vi "Process_data.vi"(0 "PWA Binary":i16[][](array[numeric]), 1 "Analogue Binary":i16[][](array[numeric]), 2 "LDA Binary output":u16[][](array[numeric]), 3 "Analogue volts":dbl[][](array[numeric]) format="%.2f", 4 "Measurement top level?":bool, 5 "Block Timings":T1={"Started"=0.0, "Ended"=0.0, "Analogue Frequency Hz"=1000.0} {"Analogue Frequency Hz" format="%.2f"}) -> (6 "Vel stat display":string[][](table), 7 "First Plot data":cluster{"Xo":dbl, "Delta X":dbl, dbl[]}[](array[cluster]) {"?" format="%.2f"; "Delta X" format="%.2f"; "Xo" format="%.2f"}, 8 "Second Plot data":cluster{"Xo":dbl, "Delta X":dbl, dbl[]}[](array[cluster]) {"?" format="%.2f"; "Delta X" format="%.2f"; "Xo" format="%.2f"}, 9 "Max Measurement time up":bool)   [LabVIEW 2011]
uses:
  Controls/Block_start_and_end.ctl
  Controls/Correlation_cluster.ctl
  Controls/Inst_type.ctl
  Controls/Instrument_Array.ctl
  Globals/Meas_global.vi
  Globals/LDA_meas_global_1.vi
  Acquisition/PWA/PWAtasksGLOBAL.vi
  Globals/Dynamic_call_global.ph.vi
  Globals/Plug_in_data_global.vi
  <vilib>/Analysis/NI_AALBase.lvlib
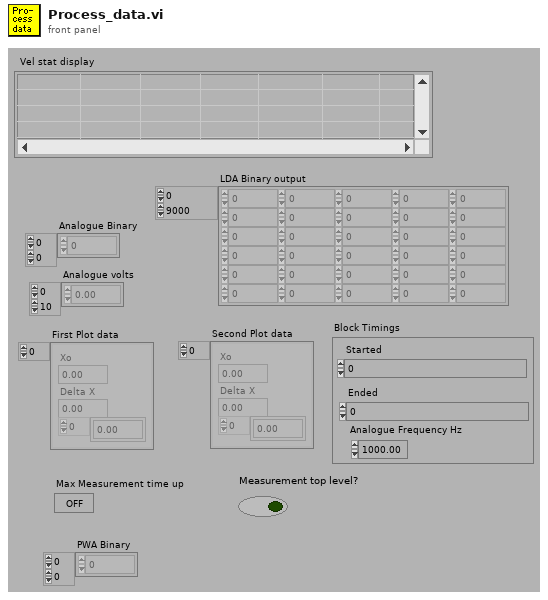
[diagram p1: front panel]
types:
  T1 = typedef "Block_start_and_end.ctl" = cluster{"Started":dbl, "Ended":dbl, "Analogue Frequency Hz":dbl}
  T2 = typedef "PWA_Data.ctl" = enum16{"No PWA Data", "One Ch PWA"}
  T3 = typedef "BSA_Type.ctl" = enum16{"57N11", "BSA F60"}
  T4 = typedef "Correlation_cluster.ctl" = cluster{"U inst":string, "W inst":string, "uw":dbl, "uw/u'w'":dbl, "u^2w":dbl, "uw^2":dbl, "uw^3":dbl, "u^3w":dbl, "u^2w^2":dbl}
  T5 = typedef "Inst_type.ctl" = enum16{"Propeller anemometer", "Raw voltage", "Pressure Transducer", "Pitot-static tube", "Preston tube", "Hot wire", "Cross wire 1", "Cross wire 2", "Generic Linear", "Generic Polynomial", "Generic BackPoly", "Fast FID", "Thermocouple", "Cold wire", "Pulsed Wire", "LDA Vel", "LDA Tran time", "LDA Arr time"}
  T6 = typedef "Instrument_Array.ctl" = enum16{"PWA", "LDA", "Analogue"}
  T7 = typedef "Analysis_info_cluster.ctl" = cluster{"Colour":u32, "Inst type":T5, "Inst name":string, "Symbol":string, "Code name":string, "Extra Info":string, "Inst Array":T6, "Index":i32, "Voltage Index":i32, "Extra Titles":string[], "Extra Values":string[], "Eng Values":dbl[], "Time (ms)":dbl[], "TT / Voltage":dbl[], "U":dbl, "u^2":dbl, "u^3":dbl, "u^4":dbl, "Skew_u":dbl, "Kurt_u":dbl, "Mean % Err":dbl, "% u'/U":dbl}
  T8 = typedef "Post_Process.ctl" = enum16{"Take New Data", "Post Process Raw Data File"}
  T9 = typedef "Graph_Type.ctl" = enum16{"Show no graph", "Voltage trace", "Velocity trace", "Vel histogram", "Spectrum", "f.E(f) v Log f", "Auto-Corr"}
  T10 = cluster{"Plot 1":u16, "Plot 2":u16, "Save graph":u16, "Plot Type":T9}
  T11 = typedef "Board_Types.ctl" = enum16{"Simulate", "Local ADAM", "Server ADAM", "NI-DAQmx", "NI-DAQmxBase", "ADC488", "DT LV-link"}
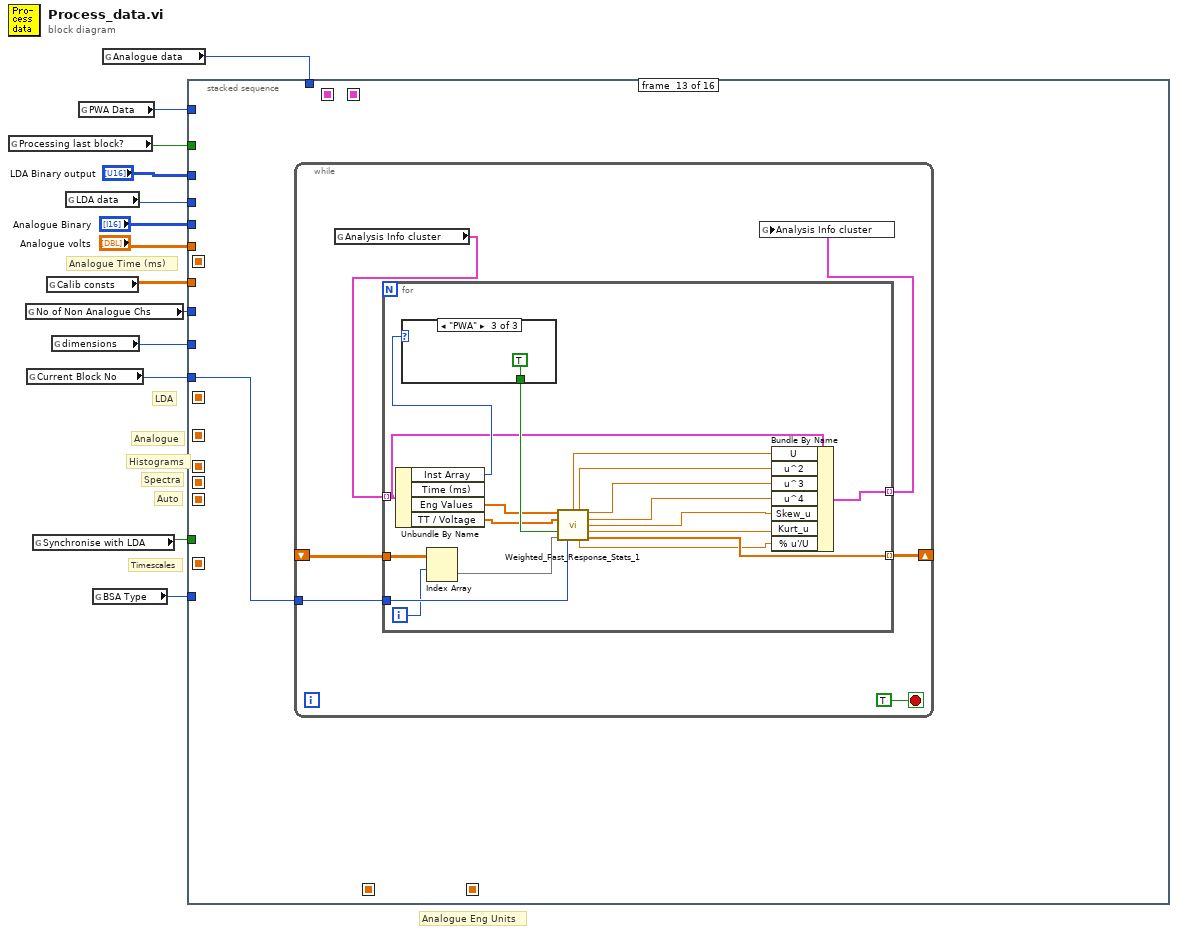
[diagram p0: block diagram]
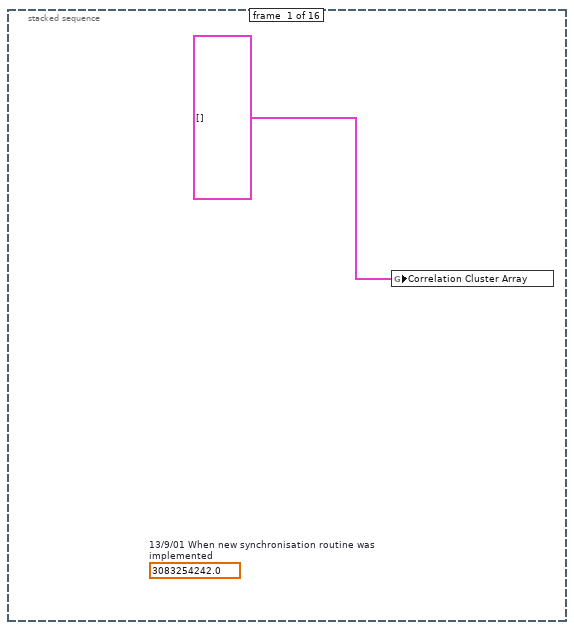
[diagram p2: hidden frame]
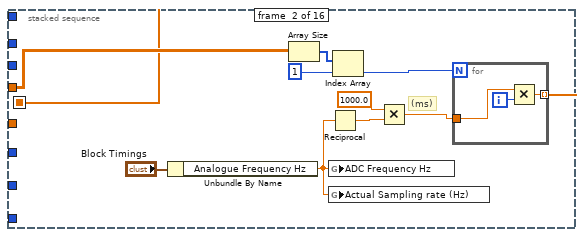
[diagram p3: hidden frame]
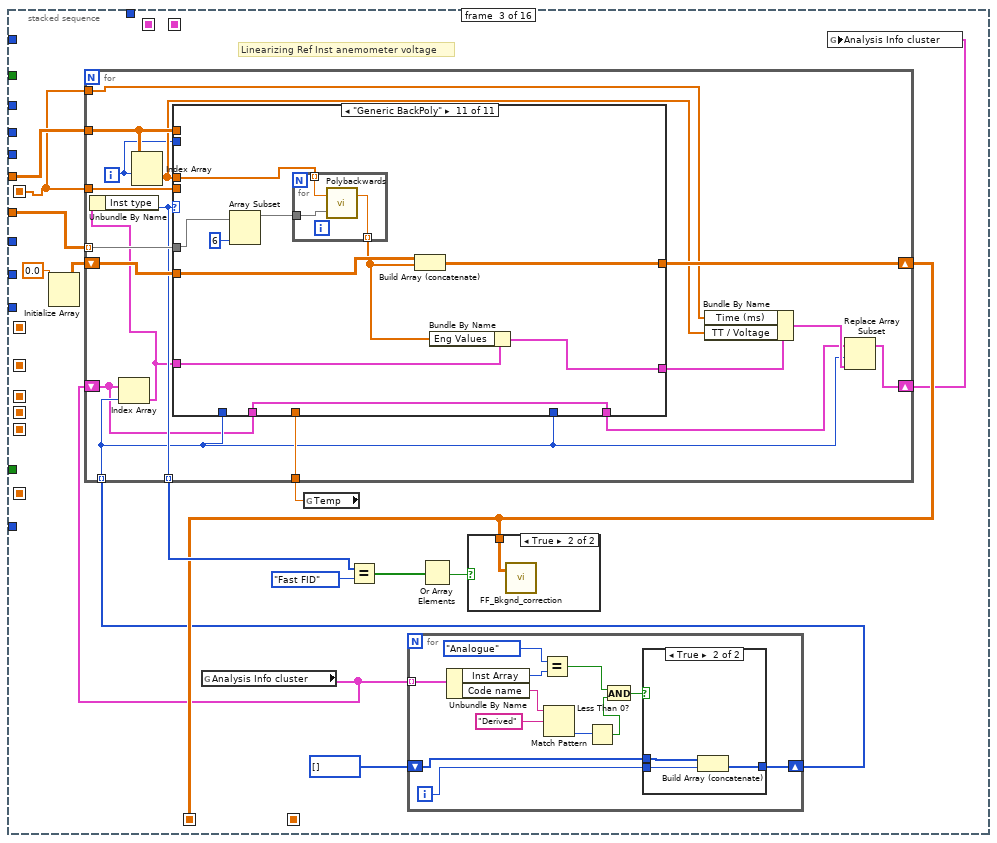
[diagram p4: hidden frame]
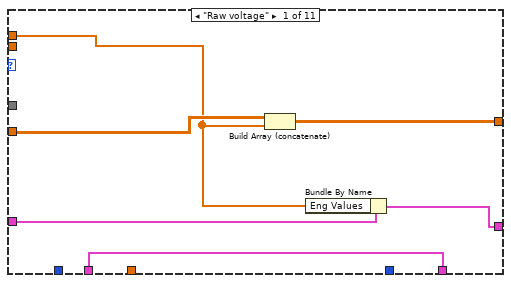
[diagram p7: hidden frame]
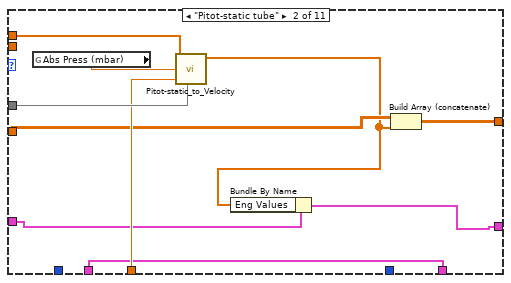
[diagram p8: hidden frame]
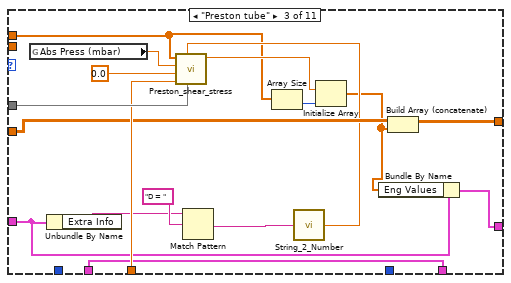
[diagram p9: hidden frame]
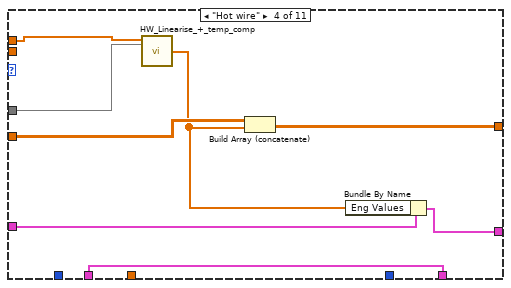
[diagram p10: hidden frame]
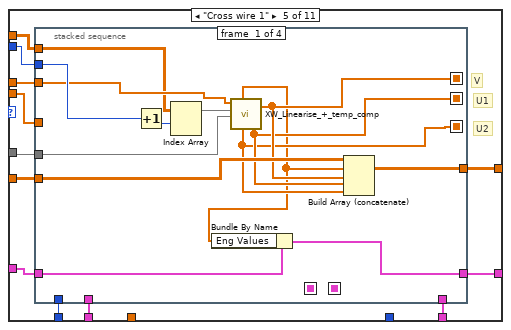
[diagram p11: hidden frame]
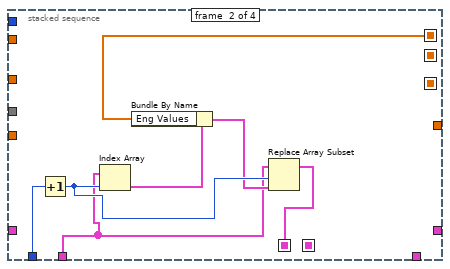
[diagram p12: hidden frame]
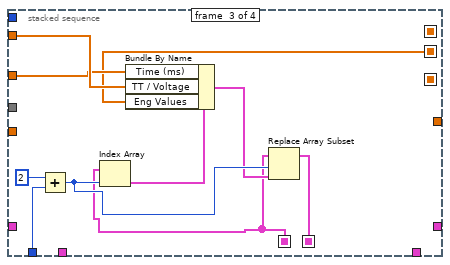
[diagram p13: hidden frame]
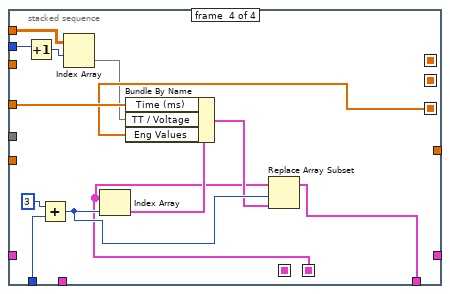
[diagram p14: hidden frame]
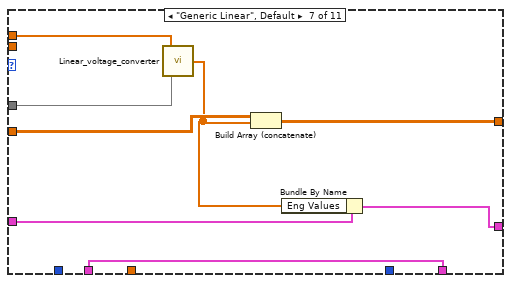
[diagram p16: hidden frame]
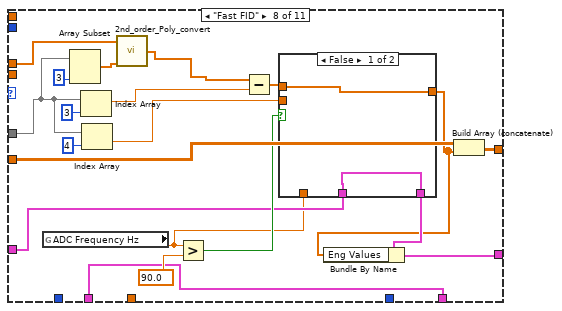
[diagram p17: hidden frame]
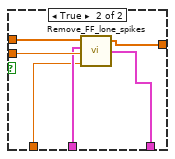
[diagram p18: hidden frame]
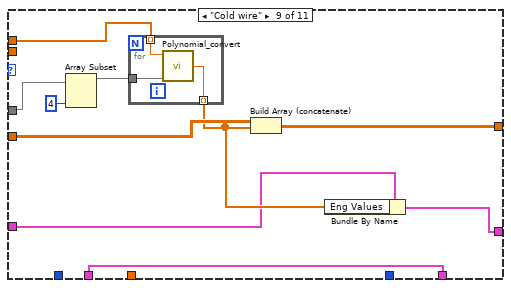
[diagram p19: hidden frame]
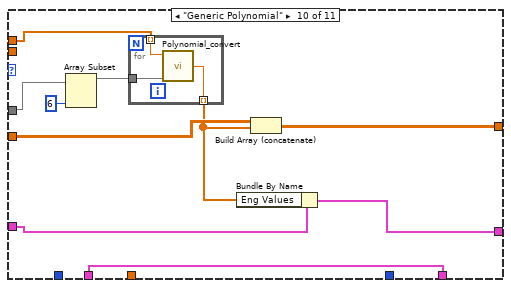
[diagram p20: hidden frame]
diagram:
  # "Analogue Time (ms)"
  # "Timescales"
  # "LDA"
  # "Auto"
  # "Spectra"
  # "Histograms"
  # "Analogue Eng Units"
  # "Analogue"
  n1 = global read "Meas_global.vi" "Processing last block?"() -> (w9:bool)
  n2 = global read "Meas_global.vi" "No of Non Analogue Chs"() -> (w5:i32)
  n3 = global read "Meas_global.vi" "Current Block No"() -> (w10:i32)
  n4 = global read "Meas_global.vi" "Synchronise with LDA"() -> (w4:bool)
  n5 = global read "Meas_global.vi" "Calib consts"() -> (w3:dbl[][])
  n6 = global read "Meas_global.vi" "dimensions"() -> (w13:enum16{"1D", "2D"})
  n7 = global read "Meas_global.vi" "LDA data"() -> (w12:enum16{"No LDA data", "Take LDA data"})
  n8 = global read "Meas_global.vi" "PWA Data"() -> (w2:T2)
  n9 = global read "LDA_meas_global_1.vi" "BSA Type"() -> (w1:T3)
  n10 = global read "Meas_global.vi" "Analogue data"() -> (w11:enum16{"No Analogue data", "Take Analogue data"})
  n11 = stacked-sequence {
    seq-local: [_ _ _ _ w278 _ _ _ _ _ _ _ _ _ _ _] -> [_ _ _ _ _ _ w545 w558 w566 w581 w592 w611 _ w644 _ _]
    seq-local: [_ _ _ w253 _ _ _ _ _ _ _ _ _ _ _ _] -> [_ _ _ _ w280 _ _ _ _ _ _ _ _ _ _ _]
    seq-local: [_ _ _ _ _ _ w544 _ _ _ _ _ _ _ _ _] -> [_ _ _ _ _ _ _ _ _ w580 _ _ _ _ w687 _]
    seq-local: [_ _ _ _ _ _ _ w557 _ _ _ _ _ _ _ _] -> [_ _ _ _ _ _ _ _ _ w579 _ _ _ _ _ _]
    seq-local: [_ _ _ _ _ _ _ _ w565 _ _ _ _ _ _ _] -> [_ _ _ _ _ _ _ _ _ w578 w599 _ _ _ _ _]
    seq-local: [_ _ _ _ _ _ _ _ _ w573 _ _ _ _ _ _] -> [_ _ _ _ _ _ _ _ _ _ _ _ _ w650 _ _]
    seq-local: [_ _ _ _ _ _ _ _ _ w572 _ _ _ _ _ _] -> [_ _ _ _ _ _ _ _ _ _ _ _ _ w649 _ _]
    seq-local: [_ _ _ _ w275 _ _ _ _ _ _ _ _ _ _ _] -> [_ _ _ _ _ _ w546 _ _ w571 _ w612 _ w645 _ w700]
    seq-local: [_ _ _ _ _ _ _ _ _ _ w585 _ _ _ _ _] -> [_ _ _ _ _ _ _ _ _ _ _ w609 _ _ _ w699]
    seq-local: [_ _ w33 _ _ _ _ _ _ _ _ _ _ _ _ _] -> [_ _ _ w252 _ _ _ _ _ _ _ _ _ _ _ _]
    seq-local: [_ w18 _ _ _ _ _ _ _ _ _ _ _ _ _ _] -> [_ _ w28 _ _ _ _ _ _ _ _ _ _ _ _ _]
    tunnel: w10 -> [_ _ _ _ _ w444 _ _ _ _ _ _ w613 _ _ _]
    tunnel: w13 -> [_ _ _ _ w282 _ _ _ _ _ _ _ _ _ _ _]
    tunnel: w12 -> [_ _ _ _ w281 _ _ _ _ _ _ _ _ _ _ _]
    tunnel: w11 -> [_ _ _ _ w279 _ _ _ _ _ _ _ _ _ _ _]
    tunnel: w9 -> [_ _ _ _ _ _ _ _ _ _ _ _ _ _ w688 _]
    tunnel: "LDA Binary output" -> [_ _ _ _ w277 _ _ _ _ _ _ _ _ w648 _ _]
    tunnel: "Analogue Binary" -> [_ _ _ _ w272 _ _ _ _ _ _ _ _ w647 w686 _]
    tunnel: "Analogue volts" -> [_ w23 w39 _ w271 _ _ _ _ w570 _ _ _ w646 w681 _]
    tunnel: w5 -> [_ _ _ _ _ _ _ _ _ _ _ _ _ _ _ _]
    tunnel: w4 -> [_ _ _ _ w276 _ _ _ _ _ _ _ _ _ _ _]
    tunnel: w3 -> [_ _ w38 _ _ _ _ _ _ _ _ _ _ _ _ _]
    tunnel: w2 -> [_ _ _ _ _ w448 _ _ _ _ _ _ _ _ _ _]
    tunnel: w1 -> [_ _ _ _ w270 _ _ _ _ _ _ _ _ _ _ _]
    frame #0 {
      (unwired) 3083254242.0  # 13/9/01 When new synchronisation routine was implemented
      n12 = global write "Meas_global.vi" "Correlation Cluster Array"(T4[] [] ("Correlation Cluster Array")) -> ()
    }
    frame #1 {
      # "(ms)"
      n13 = Unbundle By Name("Block Timings") -> ("Analogue Frequency Hz"=w19:dbl)
      n14 = Array Size(array=w23) -> (size(s)=w22:i32[])
      n15 = global write "LDA_meas_global_1.vi" "ADC Frequency Hz"(w19) -> ()
      n16 = global write "Meas_global.vi" "Actual Sampling rate (Hz)"(w19) -> ()
      n17 = Reciprocal(x=w19) -> (1/x=w17:dbl)
      n18 = Index Array(array=w22, index=1) -> (element=w20:i32)
      n19 = Multiply(x=1000.0, y=w17) -> (x*y=w15:dbl)
      n20 = for {
        N: w20 -> [_]
        tunnel: w15 -> [w26]
        tunnel: [w25] -> w18 mode=indexing
        i -> [w27]
        n21 = Multiply(x=w26, y=w27) -> (x*y=w25:dbl)
      }
    }
    frame #2 {
      # "Linearizing Ref Inst anemometer voltage"
      n22 = Initialize Array(0.0) -> (w41:dbl[][])  [unwired: 2 out]
      n23 = global read "Meas_global.vi" "Analysis Info cluster"() -> (w30:T7[])
      n24 = global read "Meas_global.vi" "Temp"() -> (w40:dbl)
      n25 = for {
        tunnel: w30 -> [w46] mode=indexing
        shift-right: [w43] -> w29
        shift-left: i32[] [] -> [w44]
        i -> [w45]
        n26 = Unbundle By Name(w46) -> ("Inst Array"=w54:T6, "Code name"=w52:string)
        n27 = Equal?(x=Instrument_Array."Analogue" ("Inst Array"), y=w54) -> (x = y?=w48:bool)
        n28 = Match Pattern(string=w52, regular expression="Derived") -> (offset past match=w50:i32)  [unwired: 4 out]
        n29 = Less Than 0?(x=w50) -> (x < 0?=w49:bool)
        n30 = And(x=w48, y=w49) -> (x .and. y?=w47:bool)
        n31 = case shown="True" w47 {
          tunnel: w45 -> [_ w58]
          tunnel: w44 -> [w55 w57]
          tunnel: [w55 w56] -> w43
          frame False {
          }
          frame True {
            n32 = Build Array (concatenate)(w57, w58) -> (w56:i32[])
          }
        }
      }
      n33 = for {
        tunnel: w39 -> [w65]
        tunnel: w38 -> [w76] mode=indexing
        shift-right: [w74] -> w33
        shift-left: w41 -> [w75]
        tunnel: w40 -> [w73]
        tunnel: [w72] -> w36 mode=indexing
        tunnel: w29 -> [w62] mode=indexing
        shift-right: [w70] -> w32
        shift-left: w30 -> [w61]
        tunnel: w28 -> [w69]
        tunnel: w28 -> [w66]
        i -> [w63]
        n34 = Index Array(array=w61, index=w62) -> (element=w71:T7)
        n35 = Unbundle By Name(w71) -> ("Inst type"=w72:T5)
        n36 = Index Array(array=w65, index (row)=w63) -> (element=w64:dbl[])  [unwired: 1 in]
        n37 = case shown="\"Generic BackPoly\"" w72 {
          tunnel: w76 -> [_ w92 w109 w117 w126 _ w184 w196 w220 w233 w246]
          tunnel: w73 -> [_ w91 w108 _ _ _ _ _ _ _ _]
          tunnel: w63 -> [_ _ _ _ w129 _ _ _ _ _ _]
          tunnel: w65 -> [_ _ _ _ w124 _ _ _ _ _ _]
          tunnel: w75 -> [w82 w90 w107 w115 w128 w176 w182 w204 w221 w234 w247]
          tunnel: [w81 w89 w106 w116 w127 w176 w183 w191 w222 w235 w248] -> w74
          tunnel: w71 -> [w80 w85 w96 w112 w123 w175 w180 w192 w215 w228 w241]
          tunnel: w62 -> [_ _ _ _ _ _ _ _ _ _ _]
          tunnel: [w79 w84 w95 w113 w122 w175 w179 w187 w214 w226 w240] -> w68
          tunnel: w69 -> [_ _ _ _ w119 _ _ _ _ _ _]
          tunnel: w64 -> [w77 w87 w93 w110 w125 _ w177 w185 w213 w229 w242]
          tunnel: w62 -> [_ _ _ _ w121 _ _ _ _ _ _]
          tunnel: w61 -> [w78 w86 w97 w114 w120 w174 w181 w189 w217 w230 w243]
          tunnel: [w78 w86 w97 w114 w118 w174 w181 w189 w217 w230 w243] -> w60
          frame "Raw voltage" {
            n38 = Build Array (concatenate)(w82, w77) -> (w81:dbl[][])
            n39 = Bundle By Name(cluster=w80, "Eng Values"=w77) -> (w79:T7)
          }
          frame "Pitot-static tube" {
            n40 = global read "Meas_global.vi" "Abs Press (mbar)"() -> (w88:dbl)
            n41 = call "Pitot-static_to_Velocity.vi"("Pressure Trans voltage"=w87, "Atmos Press mbar  (1000)"=w88, "Temp  C  (20)"=w91, "Pressure Trans Calib const"=w92) -> ("Velocity (m/s)"=w83:dbl[])  [unwired: 1 in, 3 out]
            n42 = Bundle By Name(cluster=w85, "Eng Values"=w83) -> (w84:T7)
            n43 = Build Array (concatenate)(w90, w83) -> (w89:dbl[][])
          }
          frame "Preston tube" {
            n44 = global read "Meas_global.vi" "Abs Press (mbar)"() -> (w105:dbl)
            n45 = Unbundle By Name(w96) -> ("Extra Info"=w102:string)
            n46 = Match Pattern(string=w102, regular expression="D = " ("String to match")) -> (after substring=w103:string)  [unwired: 4 out]
            n47 = Array Size(array=w93) -> (size(s)=w99:i32)
            n48 = call "String_2_Number.vi"("Value"=w103) -> ("Numeric"=w101:dbl)
            n49 = call "Preston_shear_stress.vi"("Calib. consts"=w109, "Diam. (mm)"=w101, "Temp (C)"=w108, "Static gauge head mm H2O"=0.0 ("Static gauge press mm H2O"), "Atmos. pressure (mbars)"=w105, "Pressure transducer voltages"=w93) -> ("Mean shear stress (Pa)"=w98:dbl)  [unwired: 1 in, 3 out]
            n50 = Initialize Array(w98, w99) -> (w94:dbl[])
            n51 = Bundle By Name(cluster=w96, "Eng Values"=w94) -> (w95:T7)
            n52 = Build Array (concatenate)(w107, w94) -> (w106:dbl[][])
          }
          frame "Hot wire" {
            n53 = call "HW_Linearise_+_temp_comp.vi"("Caib const"=w117, "HW voltage"=w110) -> ("Velocity"=w111:dbl[])  [unwired: 3 in, 1 out]
            n54 = Build Array (concatenate)(w115, w111) -> (w116:dbl[][])
            n55 = Bundle By Name(cluster=w112, "Eng Values"=w111) -> (w113:T7)
          }
          frame "Cross wire 1" {
            # "U2"
            # "U1"
            # "V"
            n56 = stacked-sequence {
              seq-local: [w135 _ _ _] -> [_ w149 _ _]
              seq-local: [w134 _ _ _] -> [_ _ w151 _]
              seq-local: [w133 _ _ _] -> [_ _ _ w165]
              seq-local: [_ w144 _ _] -> [_ _ w154 _]
              seq-local: [_ _ w153 _] -> [_ _ _ w168]
              tunnel: w129 -> [w143 _ _ w164]
              tunnel: w128 -> [w141 _ _ _]
              tunnel: [w140 _ _ _] -> w127
              tunnel: w126 -> [w138 _ _ _]
              tunnel: w125 -> [w137 _ w159 _]
              tunnel: w124 -> [w136 _ _ w162]
              tunnel: w123 -> [w132 _ _ _]
              tunnel: [w130 _ _ _] -> w122
              tunnel: w121 -> [_ w150 w160 w173]
              tunnel: w120 -> [_ w145 _ _]
              tunnel: w119 -> [_ _ w158 w172]
              tunnel: [_ _ _ w167] -> w118
              frame #0 {
                n57 = Increment(x=w143) -> (x+1=w142:i32)
                n58 = Index Array(array=w136, index (row)=w142) -> (element=w139:dbl[])  [unwired: 1 in]
                n59 = call "XW_Linearise_+_temp_comp.vi"("Calib const"=w138, "XW2 voltage"=w139, "XW1 voltage"=w137) -> ("U1"=w134:dbl[], "V"=w135:dbl[], "U2"=w133:dbl[], "U"=w131:dbl[])  [unwired: 1 in]
                n60 = Bundle By Name(cluster=w132, "Eng Values"=w131) -> (w130:T7)
                n61 = Build Array (concatenate)(w141, w131, w135, w134, w133) -> (w140:dbl[][])
              }
              frame #1 {
                n62 = Increment(x=w150) -> (x+1=w147:i32)
                n63 = Index Array(array=w145, index=w147) -> (element=w148:T7)
                n64 = Bundle By Name(cluster=w148, "Eng Values"=w149) -> (w146:T7)
                n65 = Replace Array Subset(array=w145, new element=w146, index=w147) -> (w144:T7[])
              }
              frame #2 {
                n66 = Add(x=2, y=w160) -> (x+y=w156:i32)
                n67 = Index Array(array=w154, index=w156) -> (element=w157:T7)
                n68 = Bundle By Name(cluster=w157, "Time (ms)"=w158, "TT / Voltage"=w159, "Eng Values"=w151) -> (w155:T7)
                n69 = Replace Array Subset(array=w154, new element=w155, index=w156) -> (w153:T7[])
              }
              frame #3 {
                n70 = Increment(x=w164) -> (x+1=w163:i32)
                n71 = Add(x=3, y=w173) -> (x+y=w170:i32)
                n72 = Index Array(array=w162, index (row)=w163) -> (element=w161:dbl[])  [unwired: 1 in]
                n73 = Index Array(array=w168, index=w170) -> (element=w171:T7)
                n74 = Bundle By Name(cluster=w171, "Time (ms)"=w172, "TT / Voltage"=w161, "Eng Values"=w165) -> (w169:T7)
                n75 = Replace Array Subset(array=w168, new element=w169, index=w170) -> (w167:T7[])
              }
            }
          }
          frame "Cross wire 2" {
          }
          frame "Generic Linear", Default {
            n76 = call "Linear_voltage_converter.vi"("Caib const A,B"=w184, "Voltage array"=w177) -> ("Converted array"=w178:dbl[])
            n77 = Build Array (concatenate)(w182, w178) -> (w183:dbl[][])
            n78 = Bundle By Name(cluster=w180, "Eng Values"=w178) -> (w179:T7)
          }
          frame "Fast FID" {
            n79 = global read "LDA_meas_global_1.vi" "ADC Frequency Hz"() -> (w190:dbl)
            n80 = Array Subset(array=w196, length=3) -> (w195:dbl[])  [unwired: 1 in]
            n81 = Index Array(array=w196, index=3) -> (element=w202:dbl)
            n82 = Index Array(array=w196, index=4) -> (element=w198:dbl)
            n83 = call "2nd_order_Poly_convert.vi"("Calib constants"=w195, "Voltage"=w185) -> ("Eng Values"=w194:dbl[])  [unwired: 4 out]
            n84 = Greater?(x=w190, y=90.0) -> (0:w193:bool)
            n85 = Subtract(x=w194, y=w202) -> (x-y=w201:dbl[])
            n86 = case shown="False" w193 {
              tunnel: w201 -> [w206 w212]
              tunnel: [w206 w211] -> w186
              tunnel: w198 -> [_ w210]
              tunnel: w192 -> [w205 w209]
              tunnel: w190 -> [_ w208]
              tunnel: [w205 w207] -> w188
              frame False {
              }
              frame True {
                n87 = call "Remove_FF_lone_spikes.vi"("ADC Frequency Hz"=w208, "Bkgnd variance"=w210, "Analysis Info cluster"=w209, "Time Trace"=w212) -> ("Analysis Info cluster out"=w207:T7, "Filtered Time Trace"=w211:dbl[])  [unwired: 1 out]
              }
            }
            n88 = Bundle By Name(cluster=w188, "Eng Values"=w186) -> (w187:T7)
            n89 = Build Array (concatenate)(w204, w186) -> (w191:dbl[][])
          }
          frame "Cold wire" {
            n90 = Array Subset(array=w220, length=4) -> (w219:dbl[])  [unwired: 1 in]
            n91 = for {
              tunnel: w219 -> [w225]
              tunnel: w213 -> [w224] mode=indexing
              tunnel: [w223] -> w216 mode=indexing
              n92 = call "Polynomial_convert.vi"("Calib constants"=w225, "Voltage"=w224) -> ("Eng Values"=w223:dbl)  [unwired: 4 out]
            }
            n93 = Build Array (concatenate)(w221, w216) -> (w222:dbl[][])
            n94 = Bundle By Name(cluster=w215, "Eng Values"=w216) -> (w214:T7)
          }
          frame "Generic Polynomial" {
            n95 = Array Subset(array=w233, length=6) -> (w232:dbl[])  [unwired: 1 in]
            n96 = for {
              tunnel: w232 -> [w238]
              tunnel: w229 -> [w237] mode=indexing
              tunnel: [w236] -> w227 mode=indexing
              n97 = call "Polynomial_convert.vi"("Calib constants"=w238, "Voltage"=w237) -> ("Eng Values"=w236:dbl)  [unwired: 4 out]
            }
            n98 = Bundle By Name(cluster=w228, "Eng Values"=w227) -> (w226:T7)
            n99 = Build Array (concatenate)(w234, w227) -> (w235:dbl[][])
          }
          frame "Generic BackPoly" {
            n100 = Array Subset(array=w246, length=6) -> (w245:dbl[])  [unwired: 1 in]
            n101 = for {
              tunnel: w245 -> [w251]
              tunnel: w242 -> [w250] mode=indexing
              tunnel: [w249] -> w239 mode=indexing
              n102 = call "Polybackwards.vi"("Coefficients"=w251, "Y input"=w250) -> ("X output"=w249:dbl)  [unwired: 1 out]
            }
            n103 = Build Array (concatenate)(w247, w239) -> (w248:dbl[][])
            n104 = Bundle By Name(cluster=w241, "Eng Values"=w239) -> (w240:T7)
          }
        }
        n105 = Bundle By Name(cluster=w68, "Time (ms)"=w66, "TT / Voltage"=w64) -> (w67:T7)
        n106 = Replace Array Subset(array=w60, new element=w67, index=w62) -> (w70:T7[])
      }
      n107 = Equal?(x=w36, y=Inst_type."Fast FID" ("Inst type")) -> (x = y?=w35:bool[])
      n108 = Or Array Elements(Boolean array=w35) -> (logical OR=w34:bool)
      n109 = case shown="True" w34 {
        tunnel: w33 -> [_ w59]
        frame False {
        }
        frame True {
          n110 = call "FF_Bkgnd_correction.vi"("Analogue Data"=w59) -> ()  [unwired: 3 out]
        }
      }
      n111 = global write "Meas_global.vi" "Analysis Info cluster"(w32) -> ()
    }
    frame #3 {
      n112 = global read "Meas_global.vi" "Post Process"() -> (w254:T8)
      n113 = case shown="\"Post Process Raw Data File\"" w254 {
        tunnel: [w255 w261] -> w253
        tunnel: w252 -> [w255 w262]
        frame "Take New Data" {
        }
        frame "Post Process Raw Data File" {
          n114 = global read "Meas_global.vi" "Raw data file"() -> (w260:path)
          n115 = Strip Path(path=w260) -> (stripped path=w259:path)  [unwired: 1 out]
          n116 = Build Path(base path=w259, name or relative path="Plugin_Info_File.txt") -> (appended path=w256:path)
          n117 = call <vilib>:"Check if File or Folder Exists.vi"("path"=w256) -> ("file or folder exists?"=w257:bool)  [unwired: 1 in, 9 out]
          n118 = case shown="True" w257 {
            tunnel: w262 -> [w263 w269]
            tunnel: [w263 w268] -> w261
            tunnel: w256 -> [_ w266]
            frame False {
            }
            frame True {
              n119 = Read from Text File(file (use dialog)=w266) -> (text=w265:string)  [unwired: 1 in, 5 out]
              n120 = call "Get_Characters_from_string.vi"("Input string"=w265, "Variable name"="Pre_Analysis_Analogue_Plugin_Name") -> ("Value"=w264:string)  [unwired: 1 in, 1 out]
              n121 = call "Call_Pre_Analysis_An_Plugin.vi"("Analogue In"=w269, "Plugin Name"=w264) -> ("Analogue Out"=w268:dbl[][])  [unwired: 1 out]
            }
          }
        }
      }
    }
    frame #4 {
      n122 = global read "Meas_global.vi" "Actual Measurement time (min)"() -> (w274:dbl)
      n123 = case shown="\"Take LDA data\"" w281 {
        tunnel: w277 -> [_ w305]
        tunnel: [w294 w299] -> w278
        tunnel: w282 -> [_ w304]
        tunnel: w280 -> [w294 w303]
        tunnel: w279 -> [_ w302]
        tunnel: w276 -> [_ w301]
        tunnel: [dbl[][] [] w300] -> w275
        tunnel: w274 -> [w284 w298]
        tunnel: [w283 w297] -> w273
        tunnel: w272 -> [w290 _]
        tunnel: w271 -> [_ w296]
        tunnel: w270 -> [_ w295]
        frame "No LDA data" {
          n124 = Array Size(array=w290) -> (size(s)=w292:i32[])
          n125 = global read "Meas_global.vi" "Actual Sampling rate (Hz)"() -> (w289:dbl)
          n126 = Index Array(array=w292, index=1) -> (element=w288:i32)
          n127 = Divide(x=w288, y=w289) -> (x/y=w286:dbl)
          n128 = Divide(x=w286, y=60.0) -> (x/y=w285:dbl)
          n129 = Add(x=w284, y=w285) -> (x+y=w283:dbl)
        }
        frame "Take LDA data" {
          # "New Sync"
          # "LDA Data"
          n130 = stacked-sequence {
            seq-local: [_ w320 _ _ _] -> [_ _ _ w363 _]
            seq-local: [w309 _ _ _ _] -> [_ w312 w333 w359 _]
            seq-local: [_ w313 _ _ _] -> [_ _ _ w358 _]
            seq-local: [_ _ w334 _ _] -> [_ _ _ w357 _]
            tunnel: w304 -> [_ w321 _ _ _]
            tunnel: w305 -> [_ w319 _ _ _]
            tunnel: w303 -> [_ _ _ w364 _]
            tunnel: w302 -> [_ _ _ w365 _]
            tunnel: w301 -> [w310 _ _ w362 _]
            tunnel: [_ _ _ w361 _] -> w300
            tunnel: [_ _ _ w360 _] -> w299
            tunnel: w298 -> [_ _ _ _ w437]
            tunnel: [_ _ _ _ w436] -> w297
            tunnel: w296 -> [_ _ _ w356 _]
            tunnel: w295 -> [_ w311 _ _ _]
            frame #0 {
              w307 = 3083254242.0  # 13/9/01 When new synchronisation routine was implemented
              n131 = global read "Meas_global.vi" "Time Data was Aquired"() -> (w308:dbl)
              n132 = Greater?(x=w308, y=w307) -> (0:w306:bool)
              n133 = Compound Arithmetic op=AND(w310, w306) -> (w309:bool)
            }
            frame #1 {
              n134 = Array Size(array=w319) -> (size(s)=w318:i32[])
              n135 = Index Array(array=w318, index=1 ("Index")) -> (element=w316:i32)
              n136 = Greater?(x=w316, y=1) -> (0:w314:bool)
              n137 = case shown="False" w314 {
                tunnel: w319 -> [_ w331]
                tunnel: w321 -> [_ w330]
                tunnel: [w325 w328] -> w320
                tunnel: [i32[] [] ("Sync Index") w329] -> w313
                tunnel: w312 -> [_ w332]
                tunnel: w311 -> [_ _]
                frame False {
                  w323 = 0 ("Dimension Size")
                  n138 = Initialize Array(0.0, w323, w323) -> (w325:dbl[][])
                  n139 = global write "LDA_meas_global_1.vi" "Arrival times"(dbl[] [] ("Weighting array")) -> ()
                }
                frame True {
                  n140 = Not(x=w332) -> (.not. x?=w327:bool)
                  n141 = call "LDA_High_Convert_New.vi"("LDA Binary data"=w331, "dimensions"=w330, "Create Sync Index"=w327) -> ("LDA data"=w328:dbl[][], "Sync Index"=w329:i32[])  [unwired: 2 out]
                }
              }
            }
            frame #2 {
              n142 = case shown="True" w333 {
                tunnel: [-1 ("f") w337] -> w334
                frame False {
                }
                frame True {
                  n143 = global read "Meas_global.vi" "Analysis Info cluster"() -> (w336:T7[])
                  n144 = Array Size(array=w336) -> (size(s)=w342:i32)
                  n145 = Decrement(x=w342) -> (x-1=w341:i32)
                  n146 = while {
                    tunnel: w336 -> [w355] mode=indexing
                    tunnel: w341 -> [w347]
                    tunnel: [w344] -> w340
                    tunnel: [w343] -> w339
                    i -> [w346]
                    stop <- w348 stop-if-true
                    n147 = Unbundle By Name(w355) -> ("Voltage Index"=w343:i32, "Inst type"=w353:T5, "Symbol"=w351:string)
                    n148 = Equal?(x=w346, y=w347) -> (x = y?=w345:bool)
                    n149 = Equal?(x=Inst_type."Raw voltage" ("Inst type"), y=w353) -> (x = y?=w349:bool)
                    n150 = Equal?(x="Sync", y=w351) -> (x = y?=w350:bool)
                    n151 = And(x=w349, y=w350) -> (x .and. y?=w344:bool)
                    n152 = Or(x=w344, y=w345) -> (x .or. y?=w348:bool)
                  }
                  n153 = Select(t=w339, s=w340, f=-1) -> (s? t:f=w337:i32)
                }
              }
            }
            frame #3 {
              n154 = case shown="\"Take Analogue data\"" w365 {
                tunnel: w364 -> [_ w376]
                tunnel: w363 -> [w367 w375]
                tunnel: w362 -> [_ w374]
                tunnel: [w367 w373] -> w361
                tunnel: [dbl[][] [] w372] -> w360
                tunnel: w359 -> [_ w371]
                tunnel: w358 -> [_ w370]
                tunnel: w357 -> [_ w369]
                tunnel: w356 -> [_ w368]
                frame "No Analogue data" {
                }
                frame "Take Analogue data" {
                  n155 = case shown="True" w374 {
                    tunnel: w376 -> [w378 w383]
                    tunnel: [w377 w382] -> w373
                    tunnel: w375 -> [w377 w386]
                    tunnel: [w378 w381] -> w372
                    tunnel: w371 -> [_ w384]
                    tunnel: w370 -> [_ w385]
                    tunnel: w369 -> [_ w380]
                    tunnel: w368 -> [_ w379]
                    frame False {
                    }
                    frame True {
                      n156 = case shown="True" w384 {
                        tunnel: w386 -> [w392 w404]
                        tunnel: w385 -> [w389 _]
                        tunnel: w383 -> [w388 w403]
                        tunnel: [w391 w400] -> w382
                        tunnel: [dbl[][] [] w403] -> w381
                        tunnel: w380 -> [_ w399]
                        tunnel: w379 -> [_ w401]
                        frame False {
                          n157 = for {
                            tunnel: w389 -> [w395]
                            tunnel: w388 -> [w394] mode=indexing
                            tunnel: [w393] -> w387 mode=indexing
                            n158 = for {
                              tunnel: w395 -> [w398] mode=indexing
                              tunnel: w394 -> [w397]
                              tunnel: [w396] -> w393 mode=indexing
                              n159 = Index Array(array=w397, index=w398) -> (element=w396:dbl)
                            }
                          }
                          n160 = Build Array (concatenate)(w392, w387) -> (w391:dbl[][])
                        }
                        frame True {
                          n161 = case shown="0, Default" w399 {
                            tunnel: w403 -> [w421 w435]
                            tunnel: [w420 w435] -> w402
                            tunnel: w401 -> [w415 _]
                            tunnel: w399 -> [w413 _]
                            frame 0, Default {
                              # "BSA sync pulse delay"
                              n162 = global read "Meas_global.vi" "Analysis Info cluster"() -> (w411:T7[])
                              n163 = Index Array(array=w415, index (row)=w413) -> (element=w412:dbl[])  [unwired: 1 in]
                              n164 = call <vilib>:"Mean.vi"("X"=w412) -> ("mean"=w405:dbl)  [unwired: 1 out]
                              n165 = global read "Meas_global.vi" "Analogue Sampling Rate"() -> (w417:dbl)
                              n166 = global read "LDA_meas_global_1.vi" "Arrival times"() -> (w419:dbl[])
                              n167 = Reciprocal(x=w417) -> (1/x=w418:dbl)
                              n168 = call "LDA_analogue_start_time_sync_PN.vi"("Burst detect HW delay (s)"=0.008 ("Sync pulse HW delay (s)"), "Correlation peak fit method"=enum32{"Max", "Quadratic", "Gaussian"}."Quadratic", "Pulse high threshold (Volts)"=w405, "Analogue dt (s)"=w418, "Analogue LDA burst pulse array"=w412, "LDA arrival Times"=w419) -> ("LDA start time rel. to Analogue (s)"=w410:dbl)  [unwired: 2 out]
                              n169 = Multiply(x=w410, y=w417) -> (x*y=w414:dbl)
                              n170 = Array Subset(array=w421, index (col)=w414) -> (w420:dbl[][])  [unwired: 3 in]
                              n171 = Multiply(x=w410, y=1000.0) -> (x*y=w408:dbl)
                              n172 = for {
                                tunnel: w411 -> [w424] mode=indexing
                                tunnel: w408 -> [w426]
                                tunnel: [w423] -> w407 mode=indexing
                                n173 = Unbundle By Name(w424) -> ("Inst Array"=w428:T6, "Time (ms)"=w425:dbl[])
                                n174 = Equal?(x=Instrument_Array."LDA" ("Inst Array"), y=w428) -> (x = y?=w422:bool)
                                n175 = case shown="False" w422 {
                                tunnel: w426 -> [_ w434]
                                tunnel: w425 -> [_ w433]
                                tunnel: w424 -> [w429 w432]
                                tunnel: [w429 w430] -> w423
                                frame False {
                                }
                                frame True {
                                n176 = Add(x=w434, y=w433) -> (x+y=w431:dbl[])
                                n177 = Bundle By Name(cluster=w432, "Time (ms)"=w431) -> (w430:T7)
                                }
                                }
                              }
                              n178 = global write "Meas_global.vi" "Analysis Info cluster"(w407) -> ()
                            }
                            frame -1 {
                            }
                          }
                          n179 = call "Sync_Afterwards.vi"("Analogue Data"=w402, "LDA Data"=w404) -> ("Eng Values"=w400:dbl[][])  [unwired: 2 out]
                        }
                      }
                    }
                  }
                }
              }
            }
            frame #4 {
              n180 = global read "LDA_meas_global_1.vi" "Time for last Block (s)"() -> (w439:dbl)
              n181 = Divide(x=w439, y=60.0) -> (x/y=w438:dbl)
              n182 = Add(x=w437, y=w438) -> (x+y=w436:dbl)
            }
          }
        }
      }
      n183 = global write "Meas_global.vi" "Actual Measurement time (min)"(w273) -> ()
    }
    frame #5 {
      n184 = case shown="\"One Ch PWA\"" w448 {
        tunnel: "PWA Binary" -> [_ w467]
        tunnel: [w450 w463] -> w446
        tunnel: [w450 w462] -> w445
        tunnel: w444 -> [_ w458]
        tunnel: [w449 w456] -> w442
        tunnel: [w449 w455] -> w443
        tunnel: [w449 w452] -> w441
        frame "No PWA Data" {
          w449 = 0 ("y")
          w450 = dbl[][] []
        }
        frame "One Ch PWA" {
          w453 = 0 ("y")
          n185 = global read "PWAtasksGLOBAL.vi" "Probe Rotated Thro' 180"() -> (w451:bool)
          n186 = global read "PWAtasksGLOBAL.vi" "Minimum TOF Index"() -> (w461:i16)
          n187 = global read "PWAtasksGLOBAL.vi" "PWA Lookup Table"() -> (w460:dbl[])
          n188 = Equal?(x=w458, y=1) -> (x = y?=w454:bool)
          n189 = Index Array(array=w467, index (row)=0) -> (element=w466:i16[])  [unwired: 1 in]
          n190 = global read "PWAtasksGLOBAL.vi" "PWA Seconds per clock pulse"() -> (w459:dbl)
          n191 = for {
            tunnel: w466 -> [w489] mode=indexing
            tunnel: [w491] -> w465 mode=indexing
            tunnel: [w490] -> w464 mode=indexing
            tunnel: w461 -> [w488]
            tunnel: w460 -> [w487]
            tunnel: w459 -> [w486]
            shift-right: [w485] -> w456
            shift-left: _ -> [w483]
            shift-right: [w484] -> w455
            shift-left: _ -> [w482]
            tunnel: w453 -> [w481]
            tunnel: w453 -> [w480]
            tunnel: w454 -> [w477]
            tunnel: w453 -> [w474]
            shift-right: [w470] -> w452
            shift-left: _ -> [w472]
            tunnel: w451 -> [w469]
            i -> [w479]
            n192 = Equal To 0?(x=w479) -> (x = 0?=w478:bool)
            n193 = And(x=w477, y=w478) -> (x .and. y?=w473:bool)
            n194 = Select(t=w481, s=w473, f=w483) -> (s? t:f=w476:i32)
            n195 = Select(t=w480, s=w473, f=w482) -> (s? t:f=w475:i32)
            n196 = Select(t=w474, s=w473, f=w472) -> (s? t:f=w471:i32)
            n197 = case shown="-4095" w489 {
              tunnel: w489 -> [w500 _ _]
              tunnel: [w505 w538 w543] -> w491
              tunnel: [w506 w538 w543] -> w490
              tunnel: w488 -> [w504 _ _]
              tunnel: w487 -> [w502 _ _]
              tunnel: w486 -> [w499 _ _]
              tunnel: w476 -> [w498 w537 w542]
              tunnel: [w497 w536 w541] -> w485
              tunnel: [w495 w535 w540] -> w484
              tunnel: w475 -> [w496 w535 w540]
              tunnel: w471 -> [w494 w534 w539]
              tunnel: [w493 w534 w539] -> w470
              tunnel: w469 -> [w492 _ _]
              frame 0, Default {
                n198 = Absolute Value(x=w500) -> (abs(x)=w501:i16)
                n199 = Greater?(x=w501, y=w504) -> (0:w503:bool)
                n200 = case shown="True" w503 {
                  tunnel: [w511 w527] -> w506
                  tunnel: [w511 w515] -> w505
                  tunnel: w500 -> [_ w526]
                  tunnel: w502 -> [_ w523]
                  tunnel: w499 -> [_ w521]
                  tunnel: w498 -> [w510 w519]
                  tunnel: [w510 w519] -> w497
                  tunnel: w496 -> [w509 w518]
                  tunnel: [w508 w518] -> w495
                  tunnel: w494 -> [w507 w512]
                  tunnel: [w507 w513] -> w493
                  tunnel: w492 -> [_ w517]
                  frame False {
                    w511 = nan
                    n201 = Increment(x=w509) -> (x+1=w508:i32)
                  }
                  frame True {
                    n202 = To Double Precision Float(number=w526) -> (double precision float=w522:dbl)
                    n203 = Add(x=w526, y=i16 4095) -> (x+y=w524:i16)
                    n204 = Multiply(x=w521, y=w522) -> (x*y=w520:dbl)
                    n205 = Index Array(array=w523, index=w524) -> (element=w516:dbl)
                    n206 = Reciprocal(x=w520) -> (1/x=w527:dbl)
                    n207 = case shown="False" w517 {
                      tunnel: w516 -> [w531 w533]
                      tunnel: [w531 w532] -> w515
                      frame False {
                      }
                      frame True {
                        n208 = Negate(x=w533) -> (-x=w532:dbl)
                      }
                    }
                    n209 = Less Than 0?(x=w515) -> (x < 0?=w514:bool)
                    n210 = case shown="False" w514 {
                      tunnel: [w528 w530] -> w513
                      tunnel: w512 -> [w528 w529]
                      frame False {
                      }
                      frame True {
                        n211 = Increment(x=w529) -> (x+1=w530:i32)
                      }
                    }
                  }
                }
              }
              frame 4095 {
                w538 = 0.0 ("Eng Values")
                n212 = Increment(x=w537) -> (x+1=w536:i32)
              }
              frame -4095 {
                w543 = 0.0 ("Eng Values")
                n213 = Increment(x=w542) -> (x+1=w541:i32)
              }
            }
          }
          n214 = Build Array(w464) -> (w463:dbl[][])
          n215 = Build Array(w465) -> (w462:dbl[][])
        }
      }
      n216 = global write "PWAtasksGLOBAL.vi" "PWA No of Reverse samples"(w441) -> ()
      n217 = global write "PWAtasksGLOBAL.vi" "PWA No of  TOF Below Min"(w443) -> ()
      n218 = global write "PWAtasksGLOBAL.vi" "PWA No of  TOF Timeouts"(w442) -> ()
      n219 = global write "PWAtasksGLOBAL.vi" "PWA 1/TOF"(w446) -> ()
      n220 = global write "PWAtasksGLOBAL.vi" "PWA Data"(w445) -> ()
    }
    frame #6 {
      n221 = global read "Meas_global.vi" "Histogram control"() -> (w549:i32[])
      n222 = Array Size(array=w549) -> (size(s)=w548:i32)
      n223 = Greater Than 0?(x=w548) -> (x > 0?=w547:bool)
      n224 = case shown="True" w547 {
        tunnel: w546 -> [_ w553]
        tunnel: w545 -> [_ w552]
        tunnel: [w550 w551] -> w544
        frame False {
          w550 = dbl[][] []  # DBL 2D array
        }
        frame True {
          n225 = call "Multi_Histogram.vi"("Equi Spaced"=w552, "Vari Spaced"=w553) -> ("Histogram"=w551:dbl[][])  [unwired: 5 out]
        }
      }
    }
    frame #7 {
      n226 = global read "Meas_global.vi" "Spectra control"() -> (w555:i32[])
      n227 = Array Size(array=w555) -> (size(s)=w556:i32)
      n228 = Greater Than 0?(x=w556) -> (x > 0?=w554:bool)
      n229 = case shown="True" w554 {
        tunnel: w558 -> [_ w561]
        tunnel: [w559 w560] -> w557
        frame False {
          w559 = dbl[][] []  # DBL 2D array
        }
        frame True {
          n230 = call "Multi_spectra.vi"("Equi Spaced"=w561) -> ("Spectra"=w560:dbl[][])  [unwired: 6 out]
        }
      }
    }
    frame #8 {
      n231 = global read "Meas_global.vi" "Auto-Corr control"() -> (w563:i32[])
      n232 = Array Size(array=w563) -> (size(s)=w564:i32)
      n233 = Greater Than 0?(x=w564) -> (x > 0?=w562:bool)
      n234 = case shown="True" w562 {
        tunnel: w566 -> [_ w569]
        tunnel: [w567 w568] -> w565
        frame False {
          w567 = dbl[][] []  # DBL 2D array
        }
        frame True {
          n235 = call "Multi_Auto-Correlation.vi"("Velocity arrays"=w569) -> ("Auto-Corr"=w568:dbl[][])  [unwired: 6 out]
        }
      }
    }
    frame #9 {
      w574 = 2  # Plot No
      w575 = 1  # Plot No
      n236 = global read "Meas_global.vi" "First Graph"() -> (w576:T10)
      n237 = call "Plotter_data.vi"("Vari Spaced"=w571, "Plot No"=w575, "Voltages"=w570, "Equi Spaced"=w581, "Histogram"=w580, "Spectra"=w579, "Auto-correlation"=w578, "Graph"=w576) -> ("Plot data"=w573:cluster{"Xo":dbl, "Delta X":dbl, dbl[]}[])  [unwired: 7 out]
      "First Plot data" <- w573
      n238 = global read "Meas_global.vi" "Second Graph"() -> (w577:T10)
      n239 = call "Plotter_data.vi"("Vari Spaced"=w571, "Plot No"=w574, "Voltages"=w570, "Equi Spaced"=w581, "Histogram"=w580, "Spectra"=w579, "Auto-correlation"=w578, "Graph"=w577) -> ("Plot data"=w572:cluster{"Xo":dbl, "Delta X":dbl, dbl[]}[])  [unwired: 7 out]
      "Second Plot data" <- w572
    }
    frame #10 {
      n240 = global read "Meas_global.vi" "No of Non Analogue Chs"() -> (w582:i32)
      n241 = Array Size(array=w592) -> (size(s)=w593:i32[])
      n242 = Index Array(array=w593, index=0) -> (element=w584:i32)
      n243 = global read "LDA_meas_global_1.vi" "LDA Timescales"() -> (w590:dbl[])
      n244 = global read "PWAtasksGLOBAL.vi" "PWA Timescales"() -> (w589:dbl[])
      n245 = Add(x=w582, y=w584) -> (x+y=w583:i32)
      n246 = Initialize Array(nan, w583) -> (w588:dbl[])
      n247 = Build Array (concatenate)(w590, w589, w588) -> (w587:dbl[])
      n248 = Array Size(array=w599) -> (size(s)=w598:i32[])
      n249 = Index Array(array=w598, index=1) -> (element=w595:i32)
      n250 = global read "Meas_global.vi" "Analogue Sampling Rate"() -> (w596:dbl)
      n251 = global read "Meas_global.vi" "Auto-Corr control"() -> (w586:i32[])
      n252 = for {
        tunnel: w599 -> [w607] mode=indexing
        tunnel: w595 -> [w608]
        tunnel: w596 -> [w606]
        shift-right: [w605] -> w585
        shift-left: w587 -> [w604]
        tunnel: w586 -> [w602] mode=indexing
        tunnel: w582 -> [w601]
        n253 = call "Calculate_Timescales.vi"("Sampling Frequency (Hz)"=w606, "Autocorrelation length"=w608, "Autocorrelation"=w607) -> ("Time Scale estimate (s)"=w603:dbl)
        n254 = Add(x=w602, y=w601) -> (x+y=w600:i32)
        n255 = Replace Array Subset(array=w604, new element=w603, index=w600) -> (w605:dbl[])
      }
      n256 = global write "Meas_global.vi" "Timescales (s)"(w585) -> ()
    }
    frame #11 {
      n257 = call "All_stats.vi"("Timescales"=w609, "Equi Spaced"=w611, "LDA"=w612) -> ("Stats array"=w610:string[])  [unwired: 2 out]
      n258 = global write "Meas_global.vi" "Vel stats info for files"(w610) -> ()
    }
    frame #12 {
      n259 = while {
        shift-right: [w617] -> _
        shift-left: _ -> [w614]
        tunnel: w613 -> [w618]
        stop <- TRUE stop-if-true
        n260 = global read "Meas_global.vi" "Analysis Info cluster"() -> (w619:T7[])
        n261 = for {
          tunnel: w619 -> [w631] mode=indexing
          tunnel: w618 -> [w633]
          tunnel: [w632] -> w617 mode=indexing
          tunnel: [w624] -> w616 mode=indexing
          tunnel: w614 -> [w622]
          i -> [w623]
          n262 = Unbundle By Name(w631) -> ("Inst Array"=w636:T6, "Eng Values"=w635:dbl[], "TT / Voltage"=w634:dbl[])  [unwired: 1 out]
          n263 = case shown="\"PWA\"" w636 {
            tunnel: [FALSE TRUE TRUE] -> w637
            frame "Analogue" {
            }
            frame "LDA" {
            }
            frame "PWA" {
            }
          }
          n264 = Index Array(array=w622, index (row)=w623) -> (element=w621:dbl[])  [unwired: 1 in]
          n265 = call "Weighted_Fast_Response_Stats_1.vi"("U"=w635, "Weighting"=w634, "Use Weighting?"=w637, "Shift in"=w621, "Block No"=w633) -> ("U"=w630:dbl, "u^2"=w629:dbl, "u^3"=w628:dbl, "u^4"=w627:dbl, "Skew"=w626:dbl, "Kurt"=w625:dbl, "% u'/U"=w620:dbl, "Shift out"=w632:dbl[])  [unwired: 3 in]
          n266 = Bundle By Name(cluster=w631, "U"=w630, "u^2"=w629, "u^3"=w628, "u^4"=w627, "Skew_u"=w626, "Kurt_u"=w625, "% u'/U"=w620) -> (w624:T7)
        }
        n267 = global write "Meas_global.vi" "Analysis Info cluster"(w616) -> ()
      }
    }
    frame #13 {
      n268 = global read "Dynamic_call_global.ph.vi" "Per Block Plug Ins"() -> (w643:string[])
      n269 = global read "Dynamic_call_global.ph.vi" "Per Block Plug Ins Extra"() -> (w642:string[])
      n270 = Build Array (concatenate)(w643, w642) -> (w641:string[])
      n271 = stacked-sequence {
        seq-local: [w651 _] -> [_ w678]
        tunnel: w645 -> [w664 _]
        tunnel: w646 -> [w663 _]
        tunnel: w648 -> [w659 _]
        tunnel: w647 -> [w660 _]
        tunnel: w650 -> [w656 _]
        tunnel: w649 -> [w654 _]
        tunnel: w644 -> [w653 _]
        tunnel: w641 -> [w652 w677]
        frame #0 {
          n272 = global write "Plug_in_data_global.vi" "Equi Spaced"(w653) -> ()
          n273 = Array Size(array=w652) -> (size(s)=w666:i32)
          n274 = Greater Than 0?(x=w666) -> (x > 0?=w651:bool)
          n275 = case shown="True" w651 {
            tunnel: [w667 w676] -> w665
            tunnel: w664 -> [_ w676]
            tunnel: w663 -> [_ w675]
            tunnel: [w667 w675] -> w662
            tunnel: [i16[][] [] ("Analogue Binary") w674] -> w661
            tunnel: w660 -> [_ w674]
            tunnel: w659 -> [_ w673]
            tunnel: [u16[][] [] ("LDA Binary output") w673] -> w658
            tunnel: [w668 w672] -> w657
            tunnel: w656 -> [_ w672]
            tunnel: [w668 w671] -> w655
            tunnel: w654 -> [_ w671]
            frame False {
              w668 = cluster{"Xo":dbl, "Delta X":dbl, dbl[]}[] [] ("Plot data")
              w667 = dbl[][] [] ("Filtered data")
            }
            frame True {
            }
          }
          n276 = global write "Plug_in_data_global.vi" "Second Plot data"(w655) -> ()
          n277 = global write "Plug_in_data_global.vi" "Analogue Binary"(w661) -> ()
          n278 = global write "Plug_in_data_global.vi" "First Plot data"(w657) -> ()
          n279 = global write "Plug_in_data_global.vi" "LDA Binary"(w658) -> ()
          n280 = global write "Plug_in_data_global.vi" "Vari Spaced"(w665) -> ()
          n281 = global write "Plug_in_data_global.vi" "Voltages"(w662) -> ()
        }
        frame #1 {
          n282 = case shown="True" w678 {
            tunnel: w677 -> [_ w680]
            frame False {
            }
            frame True {
              n283 = call "Analyse_string_array.vi"("String array"=w680) -> ("Unique strings"=w679:string[])  [unwired: 2 out]
              n284 = call "Call_Block_plug_ins.vi"("Per Block Plug Ins"=w679) -> ()
            }
          }
        }
      }
    }
    frame #14 {
      n285 = global read "Meas_global.vi" "Board type"() -> (w682:T11)
      n286 = case shown="\"DT LV-link\"" w682 {
        tunnel: w686 -> [w690 _ _ _]
        tunnel: [w689 w692 w694 w696] -> w685
        tunnel: w681 -> [_ w691 w693 w695]
        frame "Simulate", Default {
          n287 = call "Analogue_overflow_checker.vi"("I16 data"=w690) -> ("Over/Under string"=w689:string)  [unwired: 2 out]
        }
        frame "NI-DAQmx" {
          n288 = call "Voltage_overflow_checker.vi"("Voltages"=w691) -> ("Over/Under string"=w692:string)  [unwired: 2 out]
        }
        frame "NI-DAQmxBase" {
          n289 = call "Voltage_overflow_checker.vi"("Voltages"=w693) -> ("Over/Under string"=w694:string)  [unwired: 2 out]
        }
        frame "DT LV-link" {
          n290 = call "Voltage_overflow_checker.vi"("Voltages"=w695) -> ("Over/Under string"=w696:string)  [unwired: 2 out]
        }
      }
      n291 = Empty String/Path?(string/path=w685) -> (empty?=w684:bool)
      n292 = And(x=w688, y=w684) -> (x .and. y?=w683:bool)
      n293 = case shown="True" w683 {
        tunnel: w687 -> [_ w697]
        frame False {
        }
        frame True {
          n294 = call "Clipped_Hist_Check.vi"("Histogram Array"=w697) -> ()  [unwired: 1 out]
        }
      }
    }
    frame #15 {
      n295 = call "Multi_moments_LDA+_An.vi"("Timescales"=w699, "Measurement top level?"="Measurement top level?", "Vari Spaced"=w700) -> ("Max Measurement time up"=→"Max Measurement time up":bool, "File info"=w702:string[], "Vel stat display"=w703:string[][])  [unwired: 1 in]
      "Vel stat display" <- w703
      n296 = global write "Meas_global.vi" "Vel stats info for files"(w702) -> ()
      n297 = global write "Meas_global.vi" "Vel stat display"(w703) -> ()
    }
  }
